vi "MatchSettingsToSerials.vi"(11 "Serials":string[](array[string])) -> (3 "Array":string[][](array[string]))   [LabVIEW 2013, in "main.lvlib"]
uses:
  main.lvlib
  Controls/Enum Variables.ctl
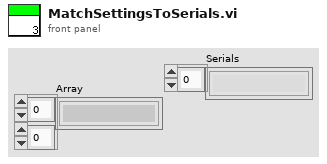
[diagram p1: front panel]
types:
  T1 = cluster{"Serial Number":string, "Side":string, "Ignore?":bool}[]
  T2 = typedef "main.lvlib/Enum Variables.ctl" = enum16{"SetAcqFilter", "GetAcqFilter", "Set Filter", "Get Filter", "Set Height", "Get Height", "Set Recorded Height", "Get Recorded Height", "Set Blue Pressure", "Get Blue Pressure", "Set Red Pressure", "Get Red Pressure", "Init", "Reset Pressure", "Set Red Cursors", "Get Red Cursors", "Set Blue Cursors", "Get Blue Cursors", "Set Language", "Get Language", "Set Active Graphs", "Get ActiveGraphs", "Set Method", "Get Method", "Set Encryption", "Get Encryption", "Set ExcelVersion", "Get ExcelVersion", "Set DICOM Avail", "Get DICOM Avail", "Set DICOM Encode", "Get DICOM Encode", "Set JournalExport", "Get JournalExport", "Set Sequence", "Get Sequence", "Set DAQ Connected", "Get DAQ Connected", "Set Current Graph", "Get Current Graph", "Set General Settings", "Get Hyphenation", "Set Arm Calc Method", "Get Arm Calc Method", "Set Dicom Tags", "Get Dicom Tags", "Set BT Serial", "Get BT Serial", "Set BT Accepted Serials", "Get BT Accepted Serials", "Get BT License", "Set BT License"}
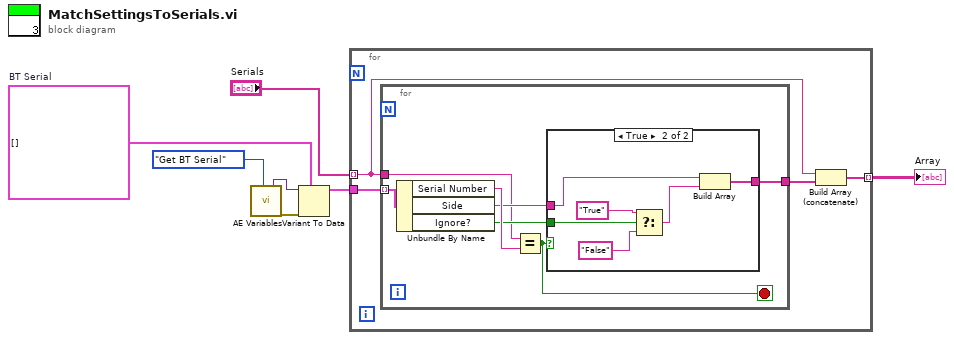
[diagram p0: block diagram]
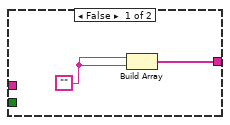
[diagram p2: hidden frame]
diagram:
  w4 = T1 []  # BT Serial
  n1 = call "AE Variables.vi"("Action"=Enum_Variables."Get BT Serial") -> ("Variant"=w5:variant, "error out"=w3:errorcluster)  [unwired: 11 in, 6 out]
  n2 = Variant To Data(error in=w3, type=w4, Variant=w5) -> (data=w6:T1)  [unwired: 1 out]
  n3 = for {
    tunnel: "Serials" -> [w10] mode=indexing
    tunnel: w6 -> [w11]
    tunnel: [w8] -> w7 mode=indexing
    n4 = for {
      tunnel: w10 -> [w13]
      tunnel: w11 -> [w18] mode=indexing
      tunnel: [w12] -> w9
      stop <- w14 stop-if-true
      n5 = Unbundle By Name(w18) -> ("Serial Number"=w17:string, "Side"=w16:string, "Ignore?"=w15:bool)
      n6 = Equal?(x=w13, y=w17) -> (x = y?=w14:bool)
      n7 = case shown="True" w14 {
        tunnel: w16 -> [_ w26]
        tunnel: w15 -> [_ w25]
        tunnel: [w19 w21] -> w12
        frame False {
          w20 = ""
          n8 = Build Array(w20, w20) -> (w19:string[])
        }
        frame True {
          n9 = Select(t="True", s=w25, f="False") -> (s? t:f=w22:string)
          n10 = Build Array(w26, w22) -> (w21:string[])
        }
      }
    }
    n11 = Build Array (concatenate)(w10, w9) -> (w8:string[])
  }
  "Array" <- w7
